vi "Stop.vi"(8 "error in (no error)":errorcluster, 10 "Message in":refnum<class "StopMessage.lvclass">, 11 "focus in":refnum<class "focus.lvclass">) -> (0 "error out":errorcluster, 3 "focus out":refnum<class "focus.lvclass">)   [LabVIEW 2012, in "focus.lvclass"]
doc: "This member function is called when the statemachine in the run.vi receives an 'stop' command. It relays the message to all observers of the component.\n\nOverride this member function in your derived class if you need additional stop functionality (but don't forget to call the parent method)."
uses:
  focus.lvclass
  <vilib>/Distrio/Murmex/StopMessage/StopMessage.lvclass
  <vilib>/Distrio/Murmex/Murmex/Murmex.lvclass
  <vilib>/Distrio/Murmex/GenericMessage/GenericMessage.lvclass
  <vilib>/Distrio/Murmex/Message/Add or replace parameter.vi
panel:
  out "Controller error":bool
  # "This method is called when the STOP\ntrigger is sent. \n\nOverride this method when your component needs to\nrespond to this trigger. \n\nCall parent for proper implementation"
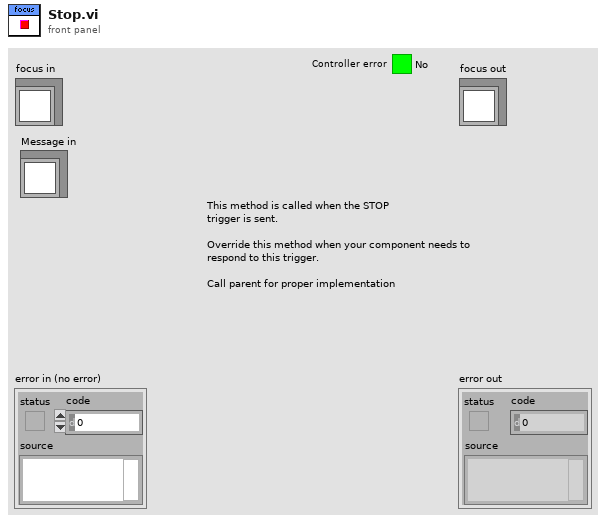
[diagram p1: front panel]
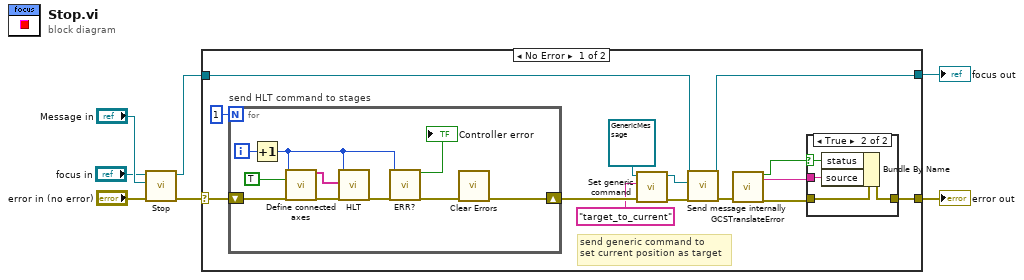
[diagram p0: block diagram]
diagram:
  n1 = call-parent "Stop.vi"("error in (no error)"="error in (no error)", "Message in"="Message in", "Murmex in"="focus in") -> ("error out"=w4:errorcluster, "Murmex out"=w2:refnum<class "focus.lvclass">)  [unwired: 7 in]
  n2 = case shown="No Error" w4 {
    selector: w4 -> [w20 w38]
    tunnel: [w18 w38] -> w3
    tunnel: w2 -> [w12 w37]
    tunnel: [w11 w37] -> w1
    frame No Error {
      # "send generic command to\nset current position as target"
      n3 = for "send HLT command to stages" {
        N: 1 -> [_]
        shift-right: [w31] -> w15
        shift-left: w20 -> [w35]
        i -> [w36]
        n4 = Increment(x=w36) -> (x+1=w28:i32)
        n5 = call "Define connected axes.vi"("System no."=w28, "Read from\ncontroller?"=TRUE ("Read from\ncontroller?"), "error in"=w35) -> ("Conn. Axes out"=w29:string[], "error out"=w34:errorcluster)  [unwired: 15 in]
        n6 = call "HLT.vi"("System no."=w28, "Affected axes"=w29, "error in"=w34) -> ("error out"=w33:errorcluster)  [unwired: 16 in]
        n7 = call "ERR?.vi"("System no."=w28, "error in"=w33) -> ("Controller error"=→"Controller error":bool, "error out"=w32:errorcluster)  [unwired: 16 in]
        n8 = call <vilib>:"Clear Errors.vi"("error in (no error)"=w32) -> ("error out"=w31:errorcluster)  [unwired: 6 in]
      }
      n9 = call <vilib>:"Set generic command.vi"("error in (no error)"=w15, "generic command"="target_to_current", "GenericMessage in"=refnum<class "GenericMessage.lvclass"> refnum ("Distrio Murmex 1.5:GenericMessage")) -> ("error out"=w14:errorcluster, "GenericMessage out"=w9:refnum<class "GenericMessage.lvclass">)  [unwired: 7 in]
      n10 = call <vilib>:"Send message internally.vi"("error in (no error)"=w14, "Message"=w9, "Murmex in"=w12) -> ("error out"=w13:errorcluster, "Murmex out"=w11:refnum<class "focus.lvclass">)  [unwired: 7 in]
      n11 = call "GCSTranslateError.vi"("error in"=w13) -> ("GCS Error?"=w17:bool, "Error Description"=w16:string, "error out"=w19:errorcluster)  [unwired: 16 in]
      n12 = case shown="True" w17 {
        selector: w17 -> [_ w24]
        tunnel: w19 -> [w22 w26]
        tunnel: [w22 w25] -> w18
        tunnel: w16 -> [_ w23]
        frame False {
        }
        frame True {
          n13 = Bundle By Name(cluster=w26, "status"=w24, "source"=w23) -> (w25:errorcluster)
        }
      }
    }
    frame Error {
    }
  }
  "error out" <- w3
  "focus out" <- w1
